vi "SeCrTS-Obtain notifier display.vi"() -> (3 "NOT DIS Out":T1)   [LabVIEW 2022 SP3]
uses:
  Control/SeCrTS-Notifier Ref.ctl
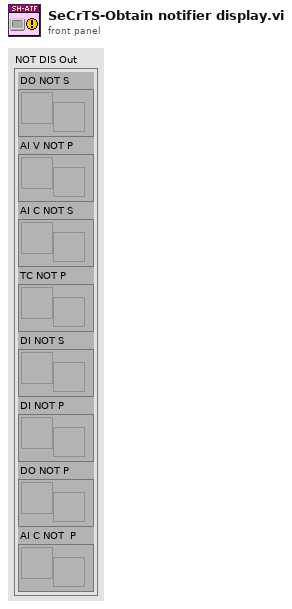
[diagram p1: front panel]
types:
  T1 = typedef "SeCrTS-Notifier Ref.ctl" = cluster{"DO NOT S":refnum<notifier>, "AI V NOT P":refnum<notifier>, "AI C NOT S":refnum<notifier>, "TC NOT P":refnum<notifier>, "DI NOT S":refnum<notifier>, "DI NOT P":refnum<notifier>, "DO NOT P":refnum<notifier>, "AI C NOT  P":refnum<notifier>}
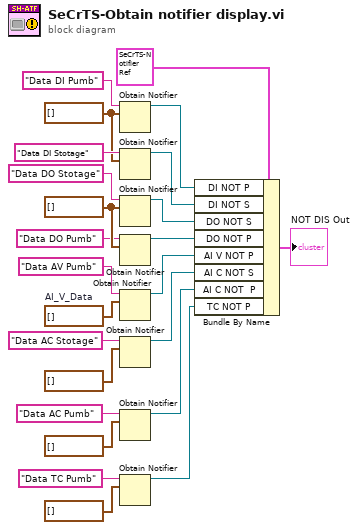
[diagram p0: block diagram]
diagram:
  w8 = digitalwaveform[] [] ("DI_Data")
  w6 = waveform(dbl)[] [] ("AI_C_Data")
  w23 = waveform(dbl)[] []  # AI_V_Data
  n1 = Obtain Notifier(name (unnamed)="Data DI Pumb", notification data type=w8) -> (notifier out=w7:refnum<notifier>)  [unwired: 2 in, 2 out]
  n2 = Obtain Notifier(name (unnamed)="Data DI Stotage", notification data type=w8) -> (notifier out=w10:refnum<notifier>)  [unwired: 2 in, 2 out]
  n3 = Obtain Notifier(name (unnamed)="Data DO Stotage", notification data type=w6) -> (notifier out=w15:refnum<notifier>)  [unwired: 2 in, 2 out]
  n4 = Obtain Notifier(name (unnamed)="Data DO Pumb", notification data type=w6) -> (notifier out=w4:refnum<notifier>)  [unwired: 2 in, 2 out]
  n5 = Obtain Notifier(name (unnamed)="Data AV Pumb", notification data type=w23) -> (notifier out=w14:refnum<notifier>)  [unwired: 2 in, 2 out]
  n6 = Obtain Notifier(name (unnamed)="Data AC Stotage", notification data type=waveform(dbl)[] [] ("AI_C_Data")) -> (notifier out=w13:refnum<notifier>)  [unwired: 2 in, 2 out]
  n7 = Obtain Notifier(name (unnamed)="Data AC Pumb", notification data type=waveform(dbl)[] [] ("AI_C_Data")) -> (notifier out=w1:refnum<notifier>)  [unwired: 2 in, 2 out]
  n8 = Obtain Notifier(name (unnamed)="Data TC Pumb", notification data type=waveform(dbl)[] [] ("AI_C_Data")) -> (notifier out=w12:refnum<notifier>)  [unwired: 2 in, 2 out]
  n9 = Bundle By Name(cluster=T1 {"DO NOT S"=refnum, "AI V NOT P"=refnum, "AI C NOT S"=refnum, "TC NOT P"=refnum, "DI NOT S"=refnum, "DI NOT P"=refnum, "DO NOT P"=refnum, "AI C NOT  P"=refnum}, "DI NOT P"=w7, "DI NOT S"=w10, "DO NOT S"=w15, "DO NOT P"=w4, "AI V NOT P"=w14, "AI C NOT S"=w13, "AI C NOT  P"=w1, "TC NOT P"=w12) -> (→"NOT DIS Out":T1)
